vi "MVE Is Library Under My Computer.vi"(11 "Full Path":string="/Untitled Project 1/My Computer/Untitled Library 1") -> (3 "Under My Computer?":bool)   [LabVIEW 2016]
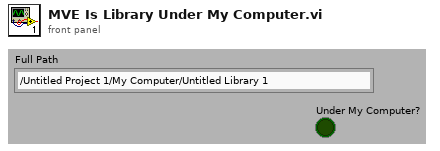
[diagram p1: front panel]
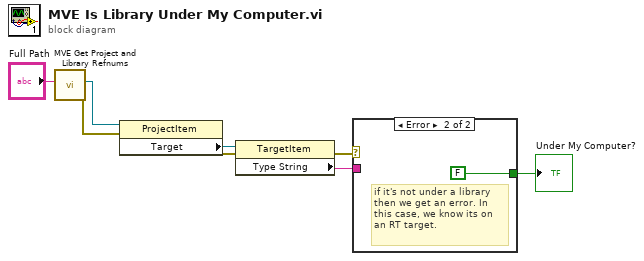
[diagram p0: block diagram]
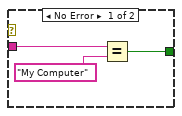
[diagram p2: hidden frame]
diagram:
  n1 = call <resource>:"MVE Get Project and Library Refnums.vi"("Full Path"="Full Path") -> ("error out"=w6:errorcluster, "ProjectItem Refnum"=w8:refnum<vi>)  [unwired: 1 in, 8 out]
  n2 = property class="ProjectItem"(reference=w8, error in=w6) -> (error out=w5:errorcluster, "Target"=w7:refnum<vi>)  [unwired: 1 out]
  n3 = property class="TargetItem"(reference=w7, error in=w5) -> (error out=w1:errorcluster, "Type String"=w3:string)  [unwired: 1 out]
  n4 = case shown="Error" w1 {
    tunnel: w3 -> [w11 _]
    tunnel: [w9 FALSE] -> w2
    frame No Error {
      n5 = Equal?(x=w11, y="My Computer") -> (x = y?=w9:bool)
    }
    frame Error {
      # "if it's not under a library\nthen we get an error. In\nthis case, we know its on \nan RT target."
    }
  }
  "Under My Computer?" <- w2
